vi "niRFUtil MT UTIL Fractional Resampler.vi"(0 "samples in":T2 format="%.2f", 5 "resampler state in":T1, 7 "offset":dbl, 9 "rate factor":dbl, 11 "error in (no error)":errorcluster, 12 "reset":bool=TRUE, 13 "flush":bool) -> (4 "samples out":T2 format="%.2f", 6 "resampler state in":T1 caption="resampler state out", 15 "error out":errorcluster)   [LabVIEW 2015, in "niRFUtil.lvlib"]
uses:
  niRFUtil.lvlib
  Includes/niRFUtil INC Complex Array.ctl
  Includes/niRFUtil MT INC Resampler State (Complex SGL).ctl
  niRFUtil MT UTIL Perform Resampling (Complex SGL).vi
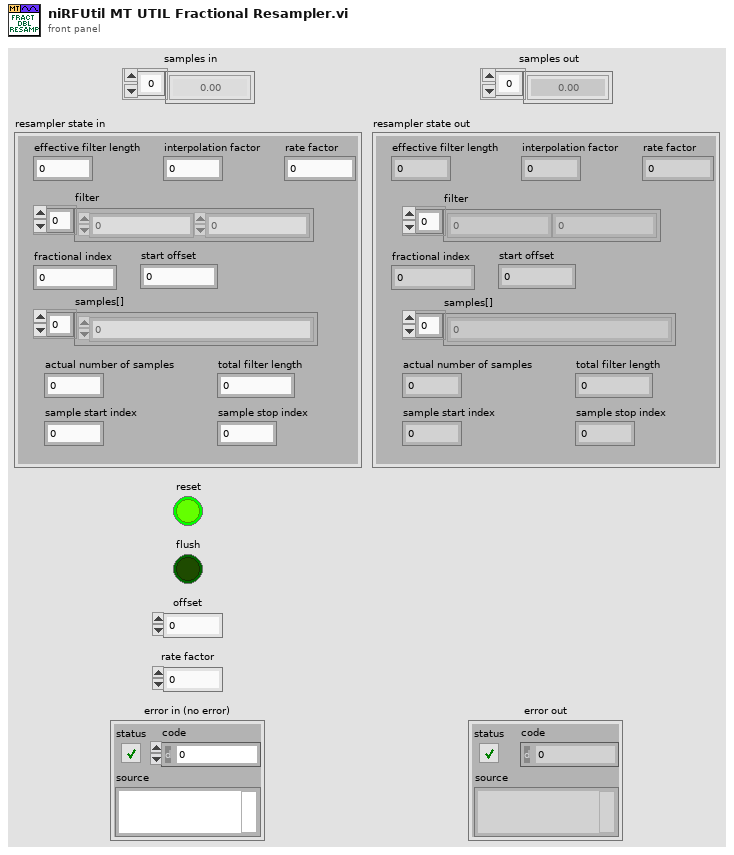
[diagram p1: front panel]
types:
  T1 = typedef "niRFUtil.lvlib/niRFUtil MT INC Resampler State (Complex SGL).ctl" = cluster{"effective filter length":i32, "interpolation factor":i32, "rate factor":dbl, "filter":sgl[], "fractional index":dbl, "start offset":i32, "samples[]":csg[], "actual number of samples":i32, "total filter length":i32, "sample start index":i32, "sample stop index":i32}
  T2 = typedef "niRFUtil.lvlib/niRFUtil INC Complex Array.ctl" = csg[]
  T3 = typedef "niRFUtil.lvlib/niRFUtil INC Real Array.ctl" = sgl[]
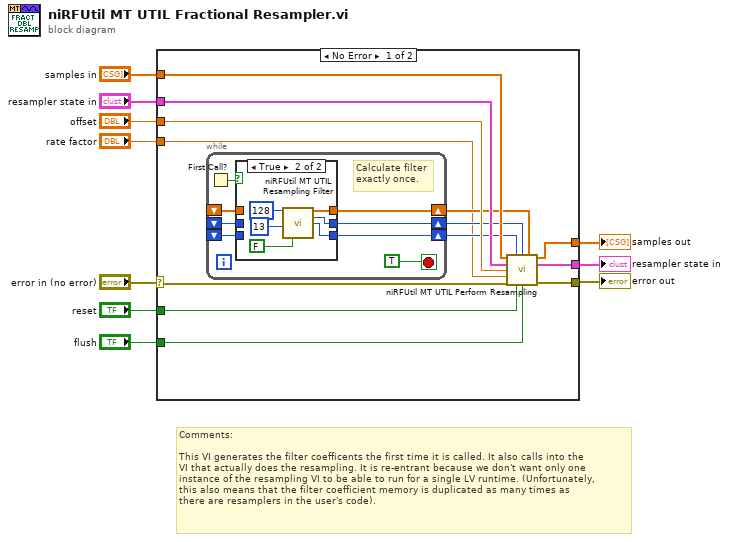
[diagram p0: block diagram]
diagram:
  # "Comments:\n\nThis VI generates the filter coefficents the first time it is called. It also calls into the\nVI that actually does the resampling. It is re-entrant because we don't want only one\ninstance of the resampling VI to be able to run for a single LV runtime. (Unfortunately,\nthis also means that the filter coefficient memory is duplicated as many times as \nthere are resamplers in the user's code)."
  n1 = case shown="No Error" "error in (no error)" {
    selector: "error in (no error)" -> [w13 w41]
    tunnel: "samples in" -> [w22 w43]
    tunnel: "resampler state in" -> [w21 w42]
    tunnel: [w20 w42] -> w8
    tunnel: "offset" -> [w17 _]
    tunnel: "reset" -> [w18 _]
    tunnel: [w19 w43] -> w5
    tunnel: [w23 w41] -> w3
    tunnel: "rate factor" -> [w11 _]
    tunnel: "flush" -> [w12 _]
    frame No Error {
      n2 = while {
        shift-right: [w31] -> w16
        shift-left: _ -> [w26]
        shift-right: [w30] -> w15
        shift-left: _ -> [w27]
        shift-right: [w29] -> w14
        shift-left: _ -> [w28]
        stop <- TRUE stop-if-true
        # "Calculate filter\nexactly once."
        n3 = First Call?() -> (First Call?: T/F=w25:bool)
        n4 = case shown="True" w25 {
          tunnel: [w32 w38] -> w31
          tunnel: [w33 w37] -> w30
          tunnel: [w34 w36] -> w29
          tunnel: w28 -> [w34 _]
          tunnel: w27 -> [w33 _]
          tunnel: w26 -> [w32 _]
          frame False {
          }
          frame True {
            n5 = call "niRFUtil MT UTIL Resampling Filter.vi"("interpolation factor in"=128, "effective filter length"=13, "legacy filter?"=FALSE) -> ("filerData[]"=w38:T3, "interpolation factor"=w37:i32, "effective filter length"=w36:i32)  [unwired: 1 in, 9 out]
          }
        }
      }
      n6 = call-poly "niRFUtil MT UTIL Perform Resampling.vi"("samples in"=w22, "effective filter length"=w14, "interpolation factor"=w15, "filterData"=w16, "resampler state in"=w21, "offset"=w17, "rate factor"=w11, "error in (no error)"=w13, "reset"=w18, "flush"=w12) -> ("samples out"=w19:csg[], "resampler state in"=w20:T1, "error out"=w23:errorcluster)  [unwired: 3 in]
    }
    frame Error {
    }
  }
  "samples out" <- w5
  "resampler state in" <- w8
  "error out" <- w3
